vi "File Initialized.vi"(8 "error in (no error)":errorcluster, 10 "Reply Payload":T1) -> (0 "error out":errorcluster)   [LabVIEW 2016, in "Logger.lvlib"]
doc: "Request the Logger to initialize the file and report when the Logger has initialized the file.\n_____\nCreated using Delacor QMH Event Scripter 4.1.0.75.\n_____\nBased on DQMH Project Template 6.1.0.94."
uses:
  Logger.lvlib
  Initialize File (Reply Payload)--cluster.ctl
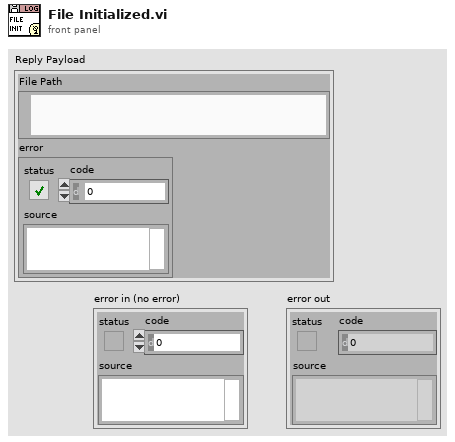
[diagram p1: front panel]
types:
  T1 = typedef "Logger.lvlib/Initialize File (Reply Payload)--cluster.ctl" = cluster{"File Path":path, "error":errorcluster}
  T2 = typedef "Logger.lvlib/Broadcast Events--cluster.ctl" = cluster{"Module Did Init":refnum<user-event>, "Status Updated":refnum<user-event>, "Error Reported":refnum<user-event>, "Module Did Stop":refnum<user-event>, "Update Module Execution Status":refnum<user-event>, "Logging Stopped":refnum<user-event>, "File Initialized":refnum<user-event>}
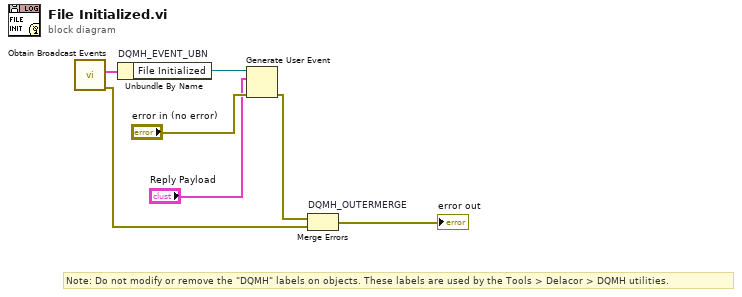
[diagram p0: block diagram]
diagram:
  # "Note: Do not modify or remove the \"DQMH\" labels on objects. These labels are used by the Tools > Delacor > DQMH utilities."
  n1 = call "Obtain Broadcast Events.vi"() -> ("error out"=w2:errorcluster, "Logger Broadcast Events"=w1:T2)  [unwired: 10 in]
  n2 = Unbundle By Name "DQMH_EVENT_UBN"(w1) -> ("File Initialized"=w4:refnum<user-event>)
  n3 = Generate User Event(user event=w4, event data cluster="Reply Payload", error in="error in (no error)") -> (error out=w3:errorcluster)  [unwired: 1 in, 1 out]
  n4 = Merge Errors "DQMH_OUTERMERGE"(w3, w2) -> (→"error out":errorcluster)
